vi "价格公式.vi"(8 "error in (no error)":errorcluster caption="错误输入（无错误）", 10 "基础价格":dbl, 11 "小杯 输入":refnum<class "小杯.lvclass">) -> (0 "error out":errorcluster caption="错误输出", 2 "价格":dbl, 3 "小杯 输出":refnum<class "小杯.lvclass">)   [LabVIEW 2016, in "小杯.lvclass"]
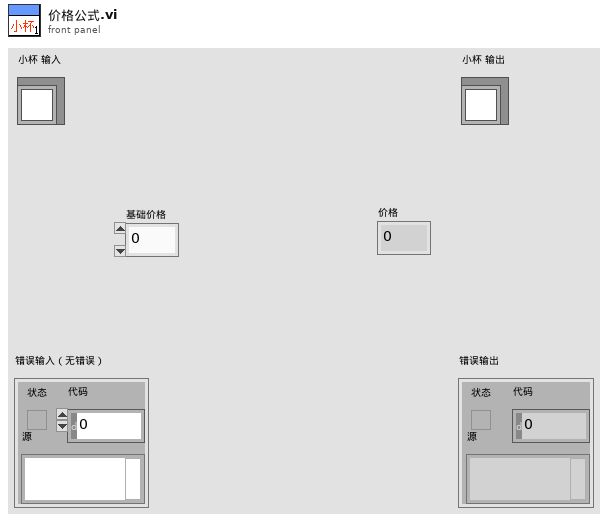
[diagram p1: front panel]
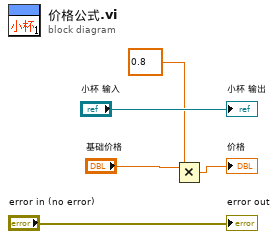
[diagram p0: block diagram]
diagram:
  n1 = Multiply(x="基础价格", y=0.8) -> (x*y=→"价格":dbl)
  "error out" <- "error in (no error)"
  "小杯 输出" <- "小杯 输入"
